vi "kDelay.vi"(8 "dimension size":i32, 11 "input":dbl) -> (3 "output":dbl)   [LabVIEW 2010, in "KevLib01.lvlib"]
uses:
  KevLib01.lvlib
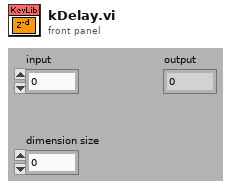
[diagram p1: front panel]
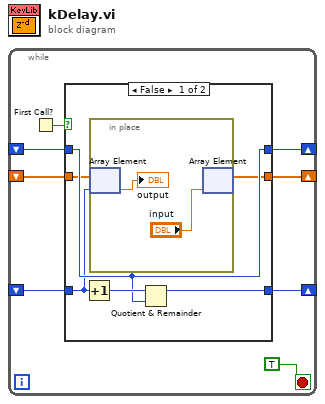
[diagram p0: block diagram]
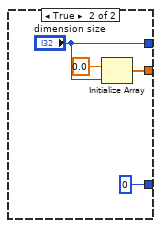
[diagram p2: hidden frame]
diagram:
  n1 = while {
    shift-right: [w6] -> _
    shift-left: _ -> [w5]
    shift-right: [w4] -> _
    shift-left: _ -> [w3]
    shift-right: [w2] -> _
    shift-left: _ -> [w1]
    stop <- TRUE stop-if-true
    n2 = First Call?() -> (First Call?: T/F=w7:bool)
    n3 = case shown="False" w7 {
      tunnel: [w13 "dimension size"] -> w6
      tunnel: w5 -> [w13 _]
      tunnel: [w9 w19] -> w4
      tunnel: w3 -> [w11 _]
      tunnel: [w12 0 ("dimension size")] -> w2
      tunnel: w1 -> [w10 _]
      frame False {
        n4 = Increment(x=w10) -> (x+1=w14:i32)
        n5 = in-place {
          n6 = in-place-array #1(w11, w10) -> (→"output":dbl)
          n7 = in-place-array #1("input") -> (w9:dbl[])  [unwired: 1 out]
        }
        n8 = Quotient & Remainder(x=w14, y=w13) -> (x-y*floor(x/y)=w12:i32)  [unwired: 1 out]
      }
      frame True {
        n9 = Initialize Array(0.0 ("element"), "dimension size") -> (w19:dbl[])
      }
    }
  }
